vi "Compression of a Metal Disk Problem.vi"() -> ()   [LabVIEW 2023]
doc: "Illustrates how to compress a metal disk when a force is applied."
uses:
  <vilib>/Analysis/1siggen.llb/Ramp Pattern by Samples.vi
  <vilib>/Analysis/polynomials.llb/1D Polynomial Evaluation (DBL).vi
  <vilib>/gmath/NI_Gmath.lvlib
  <vilib>/Analysis/NI_AALPro.lvlib
  <vilib>/Analysis/NI_AALBase.lvlib
panel:
  in  "Tab Control":enum32{"Introduction", "Calculation"}(tab)
  in  "Formulas":string[](array[string])=["(R0*sqrt(5)/H1)*((1+K*(sqrt(H0/H1)-1))*sqrt(5)-sqrt(6*H0/H1-(1+K*(sqrt(H0/H1)-1))^2))/(H1)", "-(R0*sqrt(5)/H1)*((1+K*(sqrt(H0/H1)-1))*sqrt(5)-sqrt(6*H0/H1-(1+K*(sqrt(H0/H1)-1))^2))", "R0*(1+K*(sqrt(H0/H1)-1))"]
  out "Evaluated Formulas":string[](array[string])
  in  "Force (%)":dbl(slide)=0.31797235023041476 min=0.0 max=100.0
  out "compression of a metal disk":cluster{"P(A)":dbl[], "Ramp Pattern":dbl[]}[](graph)
  in  "Stop":bool
  # "Compression is a basic process in metal forming. The face shape of the modified (under pressure) disk can usually be described by a parabolic equation where:"
  # "Here, h0 is the initial height of the body, r0 is the initial radius, h1 is the final length. The value k describes the friction coefficient (material dependent)."
  # "Overview: Demonstrates the use of the Formula Parsing and 1D & 2D Evaluation VIs to solve a parabolic equation describing the compression of a metal disk.\nRequirements: LabVIEW Full Development System\nInstructions: \n1. Run the VI. \n2. On the Calculation tab, change the Force applied to the disk and observe the result in the graph.\n3. Click Stop to stop the VI."
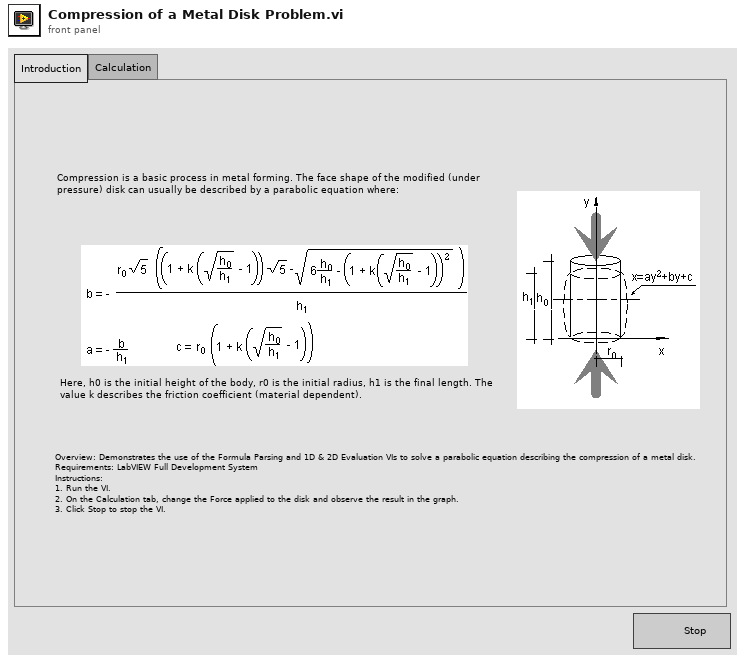
[diagram p1: front panel]
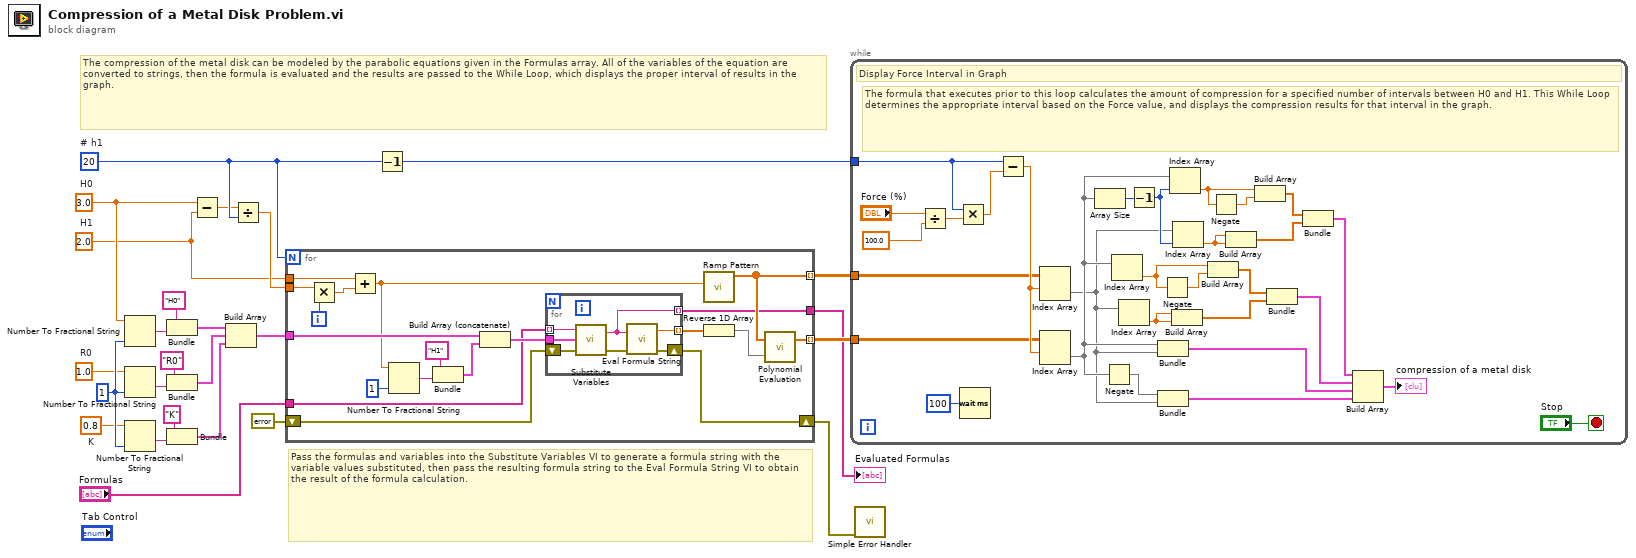
[diagram p0: block diagram]
diagram:
  w22 = 20  # # h1
  w7 = 0.8  # K
  w8 = 1.0  # R0
  w9 = 2.0  # H1
  w10 = 3.0  # H0
  w25 = i16 1 ("precision (6)")
  # "The compression of the metal disk can be modeled by the parabolic equations given in the Formulas array. All of the variables of the equation are converted to strings, then the formula is evaluated and the results are passed to the While Loop, which displays the proper interval of results in the graph."
  # "Pass the formulas and variables into the Substitute Variables VI to generate a formula string with the variable values substituted, then pass the resulting formula string to the Eval Formula String VI to obtain the result of the formula calculation."
  n1 = Number To Fractional String(number=w10, precision (6)=w25) -> (F-format string=w15:string)  [unwired: 2 out]
  n2 = Number To Fractional String(number=w8, precision (6)=w25) -> (F-format string=w18:string)  [unwired: 2 out]
  n3 = Number To Fractional String(number=w7, precision (6)=w25) -> (F-format string=w19:string)  [unwired: 2 out]
  n4 = Bundle("H0", w15) -> (w13:cluster{string, string})  [unwired: 1 out]
  n5 = Bundle("R0", w18) -> (w23:cluster{string, string})  [unwired: 1 out]
  n6 = Bundle("K", w19) -> (w24:cluster{string, string})  [unwired: 1 out]
  n7 = Subtract(x=w10, y=w9) -> (x-y=w11:dbl)
  n8 = Build Array(w13, w23, w24) -> (w12:cluster{string, string}[])
  n9 = Divide(x=w11, y=w22) -> (x/y=w16:dbl)
  n10 = for {
    N: w22 -> [_]
    tunnel: w12 -> [w41]
    tunnel: w16 -> [w37]
    tunnel: w9 -> [w36]
    tunnel: [w31] -> w5 mode=indexing
    tunnel: [w34] -> w4 mode=indexing
    tunnel: "Formulas" -> [w33]
    tunnel: [w28] -> w3
    shift-right: [w26] -> w1
    shift-left: errorcluster {"status"=FALSE, "code"=0, "source"=""} ("error constant") -> [w27]
    i -> [w44]
    n11 = Multiply(x=w37, y=w44) -> (x*y=w30:dbl)
    n12 = Add(x=w36, y=w30) -> (x+y=w32:dbl)
    n13 = Number To Fractional String(number=w32, precision (6)=i16 1) -> (F-format string=w42:string)  [unwired: 2 out]
    n14 = Bundle("H1", w42) -> (w40:cluster{string, string})  [unwired: 1 out]
    n15 = Build Array (concatenate)(w41, w40) -> (w39:cluster{string, string}[])
    n16 = for {
      tunnel: w39 -> [w51]
      tunnel: w33 -> [w50] mode=indexing
      tunnel: [w49] -> w38 mode=indexing
      tunnel: [w48] -> w28 mode=indexing
      shift-right: [w45] -> w26
      shift-left: w27 -> [w46]
      n17 = call <vilib>:"Substitute Variables.vi"("error in (no error)"=w46, "Substitution Rules"=w51, "original formula"=w50) -> ("error out"=w47:errorcluster, "formula after substitution"=w48:string)
      n18 = call <vilib>:"Eval Formula String.vi"("error in (no error)"=w47, "formula"=w48) -> ("error out"=w45:errorcluster, "y value"=w49:dbl)
    }
    n19 = call-poly <vilib>:"Ramp Pattern.vi"("end"=w32) -> ("Ramp Pattern"=w31:dbl[])  [unwired: 9 in, 1 out]
    n20 = Reverse 1D Array(array=w38) -> (reversed array=w35:dbl[])
    n21 = call-poly <vilib>:"Polynomial Evaluation.vi"("P(x)"=w35, "A"=w31) -> ("P(A)"=w34:dbl[])  [unwired: 1 out]
  }
  "Evaluated Formulas" <- w3
  n22 = Decrement(x=w22) -> (x-1=w6:i32)
  n23 = while {
    tunnel: w6 -> [w60]
    tunnel: w5 -> [w59]
    tunnel: w4 -> [w58]
    stop <- "Stop" stop-if-true
    # "The formula that executes prior to this loop calculates the amount of compression for a specified number of intervals between H0 and H1. This While Loop determines the appropriate interval based on the Force value, and displays the compression results for that interval in the graph."
    # "Display Force Interval in Graph"
    n24 = Divide(x="Force (%)", y=100.0) -> (x/y=w65:dbl)
    n25 = Multiply(x=w60, y=w65) -> (x*y=w64:dbl)
    n26 = Wait (ms)(milliseconds to wait=u32 100) -> ()  [unwired: 1 out]
    n27 = Subtract(x=w60, y=w64) -> (x-y=w63:dbl)
    n28 = Index Array(array=w59, index (row)=w63) -> (element=w57:dbl[])  [unwired: 1 in]
    n29 = Index Array(array=w58, index (row)=w63) -> (element=w70:dbl[])  [unwired: 1 in]
    n30 = Array Size(array=w70) -> (size(s)=w69:i32)
    n31 = Negate(x=w70) -> (-x=w80:dbl[])
    n32 = Index Array(array=w70) -> (element=w56:dbl)  [unwired: 1 in]
    n33 = Index Array(array=w57) -> (element=w78:dbl)  [unwired: 1 in]
    n34 = Decrement(x=w69) -> (x-1=w66:i32)
    n35 = Bundle("P(A)"=w70, "Ramp Pattern"=w57) -> (w74:cluster{"P(A)":dbl[], "Ramp Pattern":dbl[]})  [unwired: 1 out]
    n36 = Bundle(w80, "Ramp Pattern"=w57) -> (w75:cluster{dbl[], "Ramp Pattern":dbl[]})  [unwired: 1 out]
    n37 = Negate(x=w56) -> (-x=w55:dbl)
    n38 = Index Array(array=w70, index=w66) -> (element=w54:dbl)
    n39 = Build Array(w78, w78) -> (w76:dbl[])
    n40 = Index Array(array=w57, index=w66) -> (element=w53:dbl)
    n41 = Build Array(w56, w55) -> (w77:dbl[])
    n42 = Negate(x=w54) -> (-x=w71:dbl)
    n43 = Build Array(w53, w53) -> (w68:dbl[])
    n44 = Build Array(w54, w71) -> (w72:dbl[])
    n45 = Bundle(w77, w76) -> (w73:cluster{dbl[], dbl[]})  [unwired: 1 out]
    n46 = Bundle(w72, w68) -> (w67:cluster{dbl[], dbl[]})  [unwired: 1 out]
    n47 = Build Array(w67, w73, w74, w75) -> (→"compression of a metal disk":cluster{"P(A)":dbl[], "Ramp Pattern":dbl[]}[])
  }
  n48 = call <vilib>:"Simple Error Handler.vi"("error in (no error)"=w1) -> ()  [unwired: 4 in, 5 out]
